vi "GetValueAndCheckRange.vi"(4 "user error":errorcluster, 5 "config array":string[][](array[string]), 6 "Arguments":string, 7 "Command":string) -> (0 "USER error out":errorcluster, 1 "OK to change":bool, 2 "element":string, 3 "setValue":string)   [LabVIEW 2013]
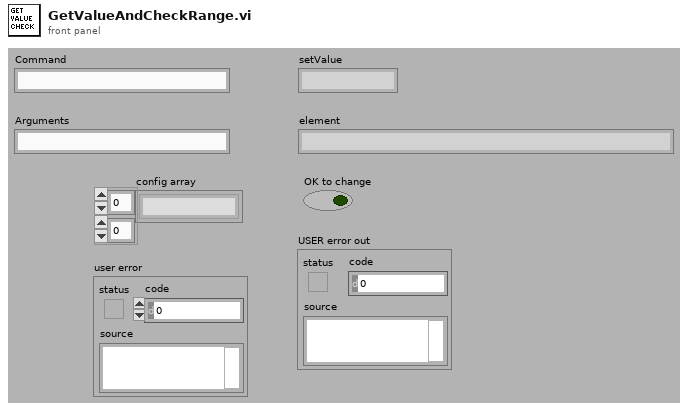
[diagram p1: front panel]
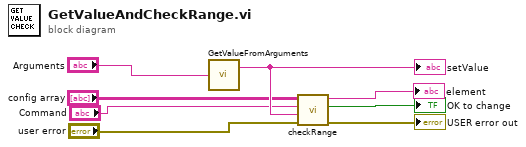
[diagram p0: block diagram]
diagram:
  n1 = call "GetValueFromArguments.vi"("Arguments"="Arguments") -> ("setValue"=w8:string)  [unwired: 1 out]
  "setValue" <- w8
  n2 = call "checkRange.vi"("USER error in"="user error", "setValue"=w8, "setcommand"="Command", "config array"="config array") -> ("USER error out"=→"USER error out":errorcluster, "OK to change"=→"OK to change":bool, "element"=→"element":string)  [unwired: 1 in]
